vi "format_data.vi"() -> ()   [LabVIEW 2020]
panel:
  out "XY Graph":cluster{dbl[], dbl[]}[](graph)
  in  "Earth":dbl[](array[numeric])
  in  "Sun":dbl[](array[numeric])
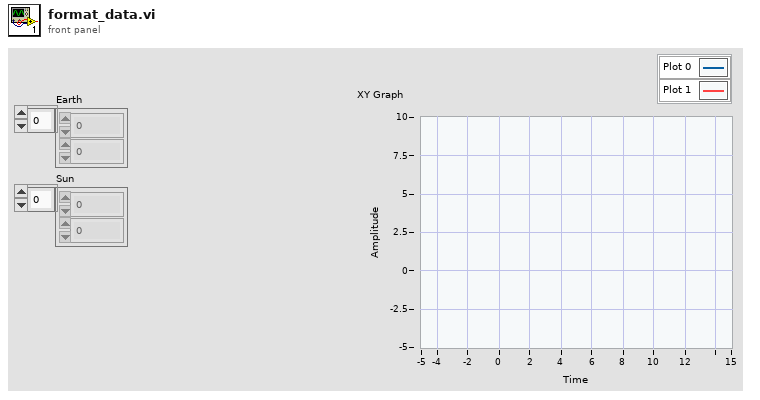
[diagram p1: front panel]
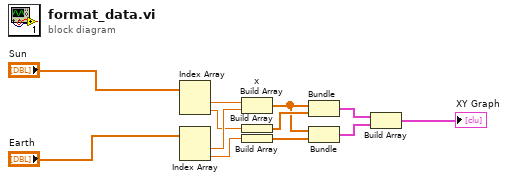
[diagram p0: block diagram]
diagram:
  n1 = Index Array(array="Sun") -> (element #1=w12:dbl, element #2=w8:dbl)  [unwired: 2 in]
  n2 = Index Array(array="Earth") -> (element #1=w11:dbl, element #2=w7:dbl)  [unwired: 2 in]
  n3 = Build Array "x"(w12, w11) -> (w5:dbl[])
  n4 = Build Array(w8) -> (w6:dbl[])
  n5 = Build Array(w7) -> (w4:dbl[])
  n6 = Bundle(w5, w6) -> (w3:cluster{dbl[], dbl[]})  [unwired: 1 in]
  n7 = Bundle(w5, w4) -> (w2:cluster{dbl[], dbl[]})  [unwired: 1 in]
  n8 = Build Array(w3, w2) -> (→"XY Graph":cluster{dbl[], dbl[]}[])
